vi "Process.vi"(8 "error in":errorcluster, 11 "Maui 2.0":refnum<class "Maui 2.0.lvclass">) -> (0 "error out":errorcluster, 3 "Maui 2.0 out":refnum<class "Maui 2.0.lvclass">)   [LabVIEW 2020, in "Maui 2.0.lvclass"]
doc: "---------------------------------------------------------------\nJKI State Machine Objects™\nhttp://jki.net/state-machine-objects/\nCopyright (C) 2005-2015, JKI <info@jki.net>\nALL RIGHTS RESERVED"
uses:
  Maui 2.0.lvclass
  C:/Program Files (x86)/National Instruments/LabVIEW 2020/vi.lib/JKI/JKI SMO/SMO/SMO.lvclass
  <vilib>/JKI/JKI SMO/SMO/Typedefs/Parent Call--Enum.ctl
  <vilib>/JKI/JKI SMO/SMO/SMO.lvclass
  Lifeguard/Lifeguard.lvclass
  Maui Manager/Maui Manager.lvclass
  Maui Manager/Maui Manager.lvclass/Maui Manager.ctl
  Maui Manager/Accessors/Write Processes.vi
  Maui Manager/Accessors/Write Panels.vi
panel:
  # "For instructions on how to use the JKI State Machine Objects, examples and video tutorials, visit:\nhttp://jki.net/state-machine-objects/\n\nJKI State Machine Objects™\nhttp://jki.net/state-machine-objects/\nCopyright (C) 2005-2015, JKI <info@jki.net>\nALL RIGHTS RESERVED"
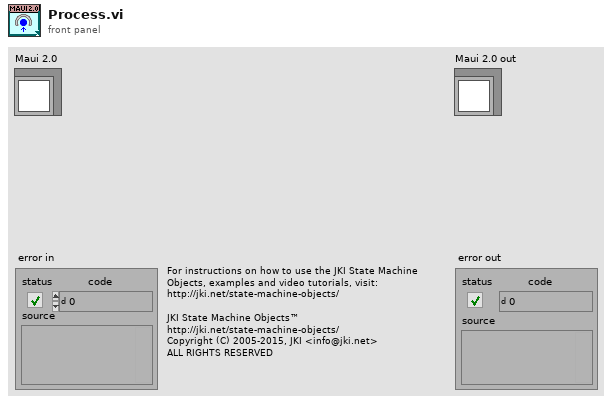
[diagram p1: front panel]
types:
  T1 = typedef "SMO.lvclass/Parent Call--Enum.ctl" = enum16{"Allows parent to run", "Does not request parent to run"}
  T2 = cluster{"Control":refnum<vi>, "Subpanel":refnum<vi>, "Active":i32, "Ctrl Class":string}
  T3 = enum32{"invalid app kind", "Development System", "Run Time System", "Student Edition", "Embedded LabVIEW", "Evaluation", "Custom"}
  T4 = enum32{"Invalid", "Standard", "Closed", "Hidden", "Minimized", "Maximized"}
  T5 = cluster{"Core":cluster{"Current VI Reference":refnum<vi>, "Close Panel on Exit?":bool, "error":errorcluster}, "Self Reference":refnum<class "Maui 2.0.lvclass">, "Subpanels":refnum<class "SMO.lvclass">[], "Panels":cluster{"Control":refnum<vi>, "Subpanel":refnum<vi>, "Active":i32, "Ctrl Class":string}[], "Lifeguard":refnum<class "Lifeguard.lvclass">, "Maui Manager":refnum<class "Maui Manager.lvclass">, "New Value":i32, "Panel":i32}
  T6 = typedef "Maui 2.0.lvclass/PrivateEvents--Maui 2.0.Set Panels.ctl" = cluster{"Control":refnum<vi>, "SubPnl":refnum<vi>}[]
  T7 = typedef "Maui 2.0.lvclass/PrivateEvents--Maui 2.0.Get Subpanels.ctl" = refnum<notifier>
  T8 = cluster{"Control":refnum<vi>, "Subpanel":refnum<vi>, "Active":i32, "Ctrl Class":string}[]
  T9 = cluster{"Current VI Reference":refnum<vi>, "Close Panel on Exit?":bool, "error":errorcluster}
  T10 = typedef "SMO.lvclass/Protected Events.ctl" = cluster{"StopProcesses":refnum<user-event>, "AbortProcesses":refnum<user-event>, "Config Changed":refnum<user-event>, "Dependency":refnum<user-event>}
  T11 = typedef "Maui 2.0.lvclass/PrivateEvents--Cluster.ctl" = cluster{"Set Subpanels":refnum<user-event>, "Get Subpanels":refnum<user-event>, "Set Panels":refnum<user-event>}
  T12 = typedef "Lifeguard.lvclass/PublicEvents--Cluster.ctl" = cluster{"New Panel Value":refnum<user-event>}
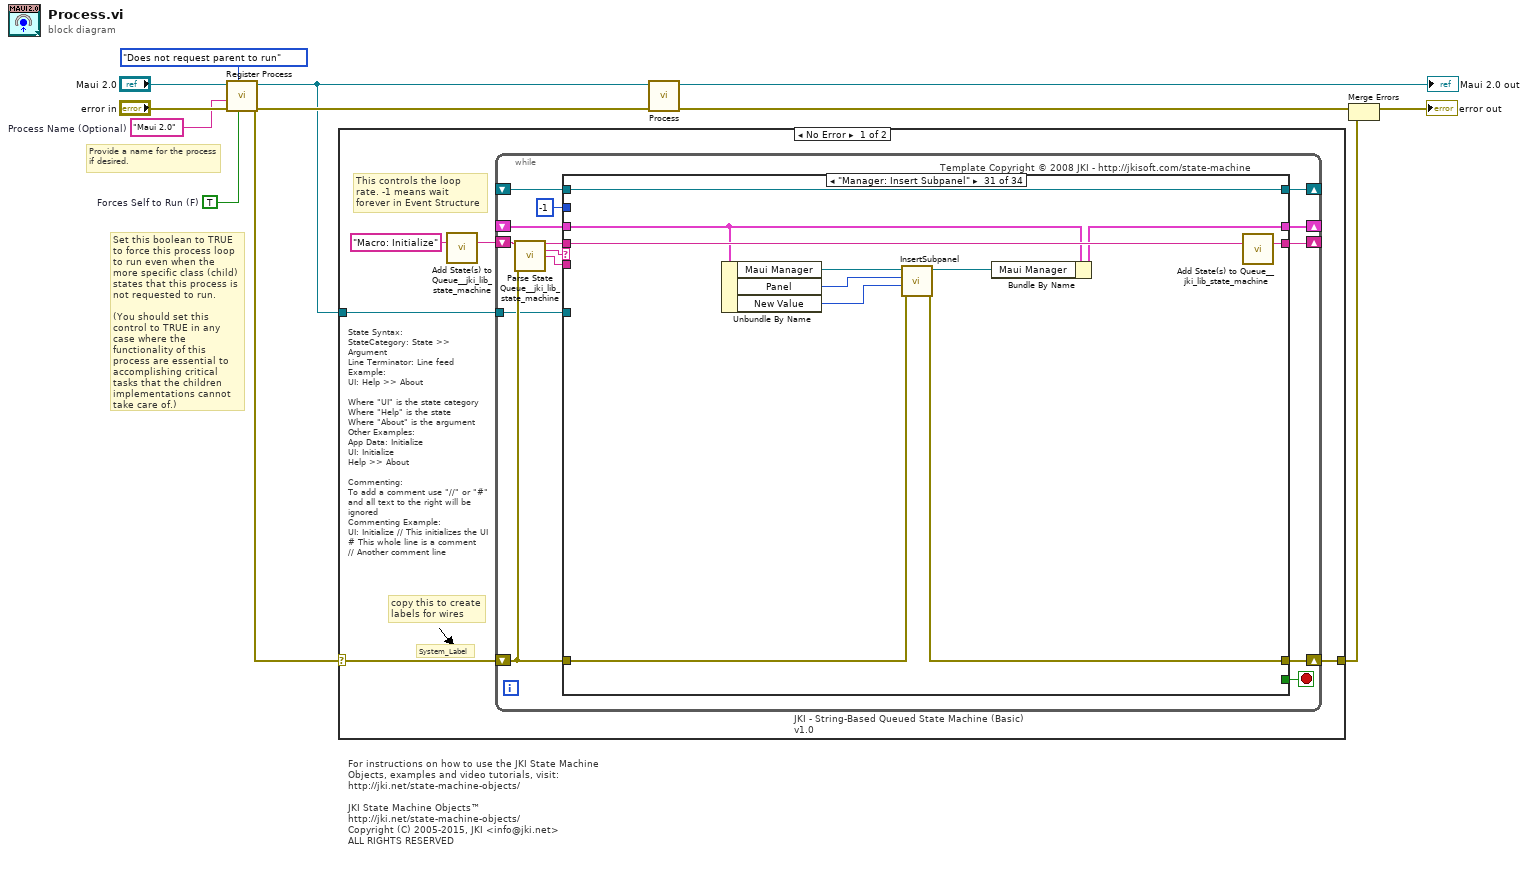
[diagram p0: block diagram]
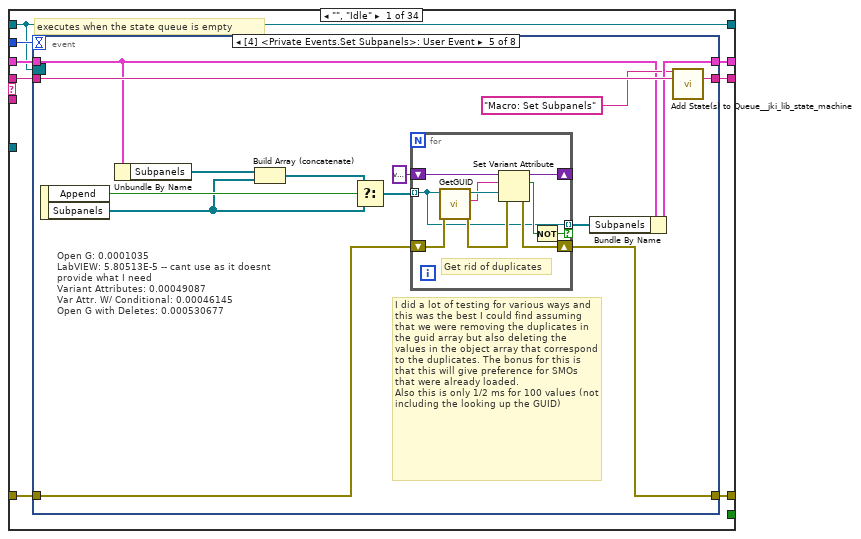
[diagram p2: hidden frame]
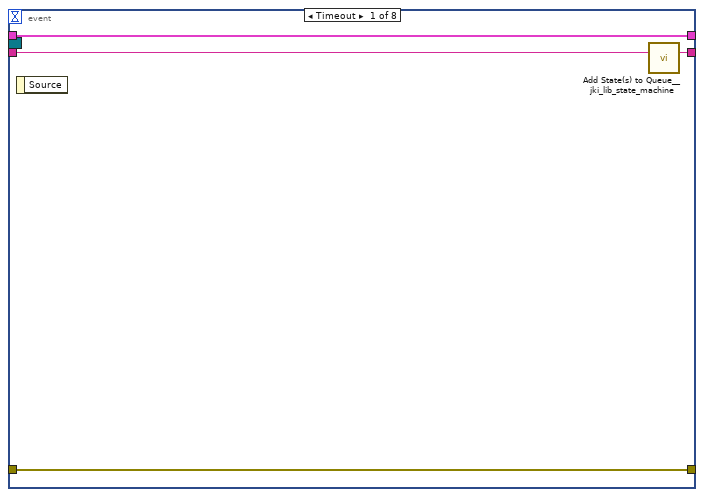
[diagram p3: hidden frame]
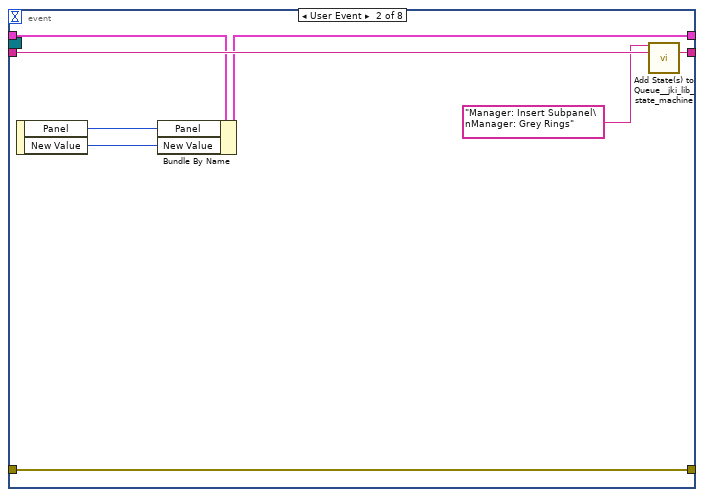
[diagram p4: hidden frame]
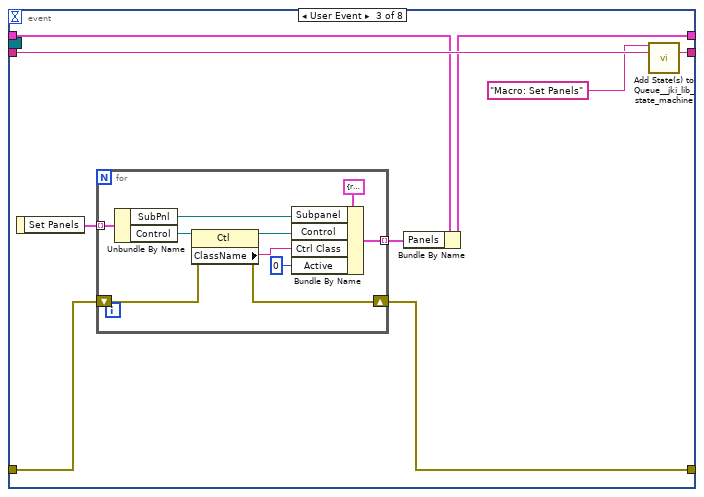
[diagram p5: hidden frame]
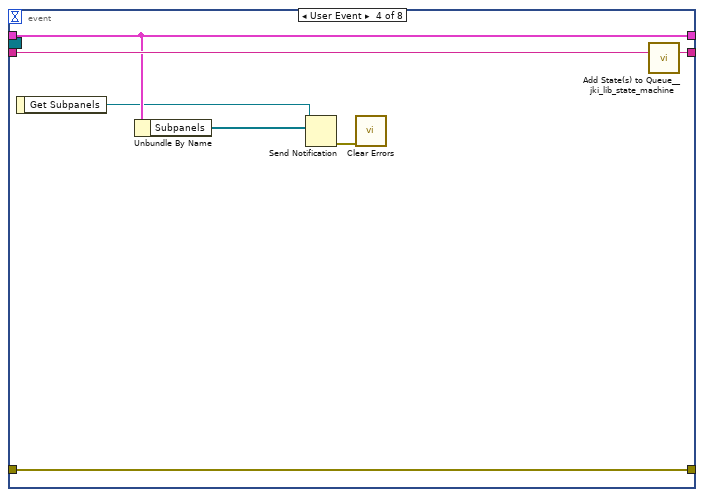
[diagram p6: hidden frame]
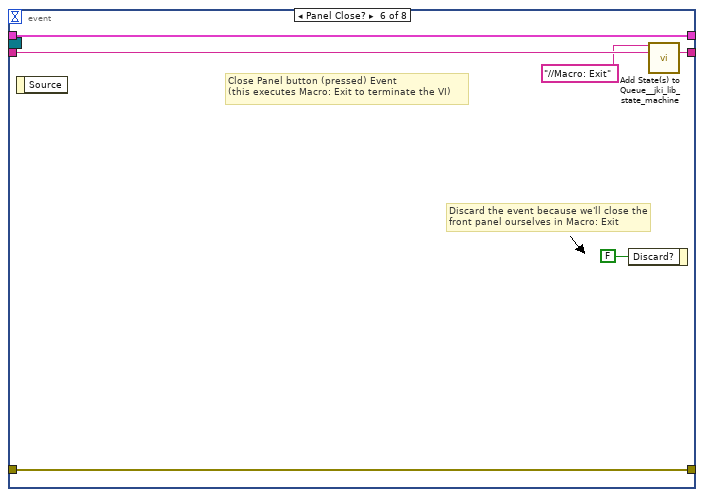
[diagram p7: hidden frame]
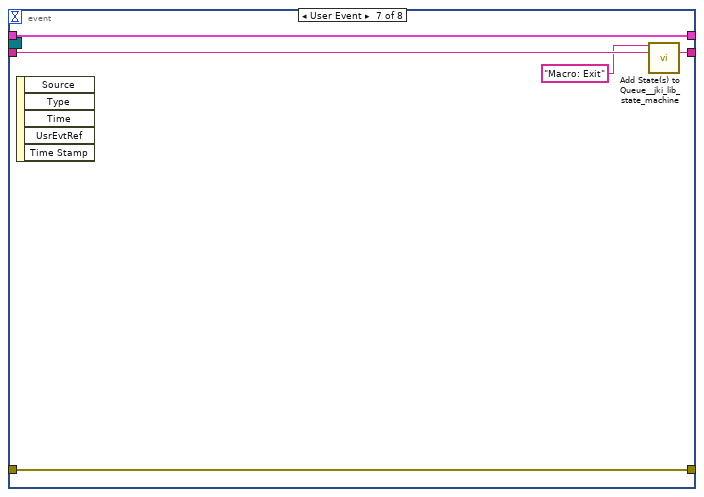
[diagram p8: hidden frame]
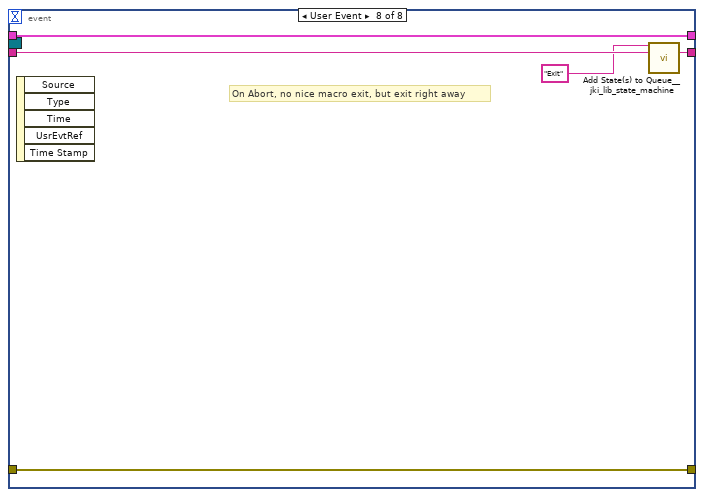
[diagram p9: hidden frame]
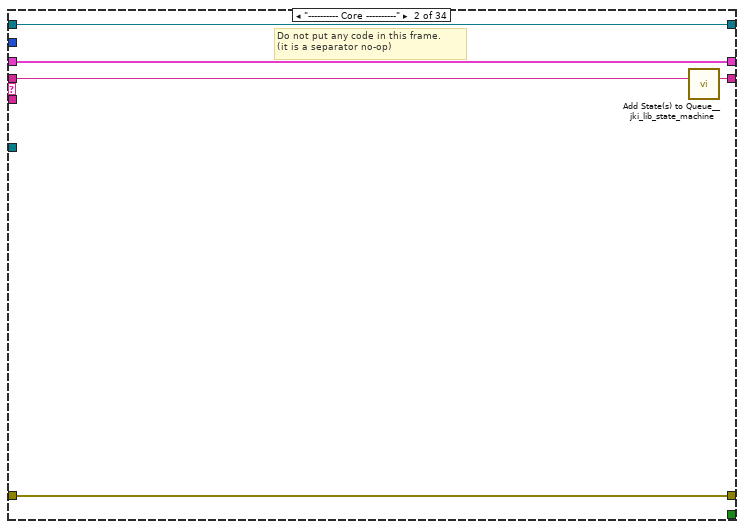
[diagram p10: hidden frame]
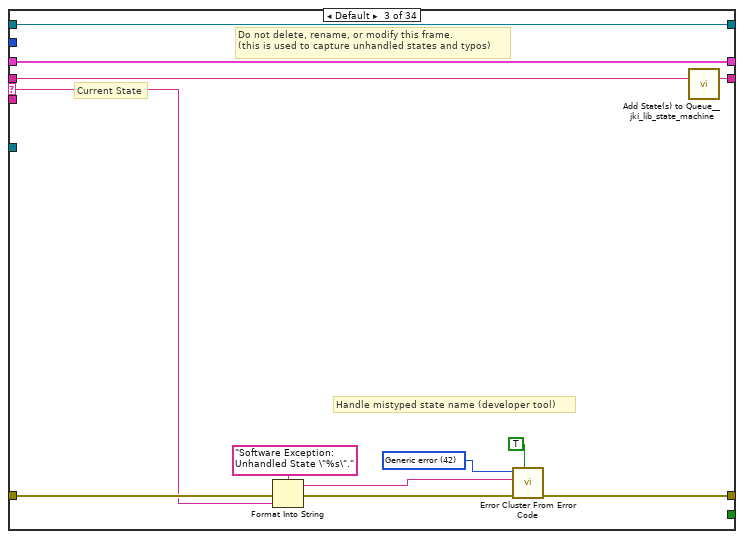
[diagram p11: hidden frame]
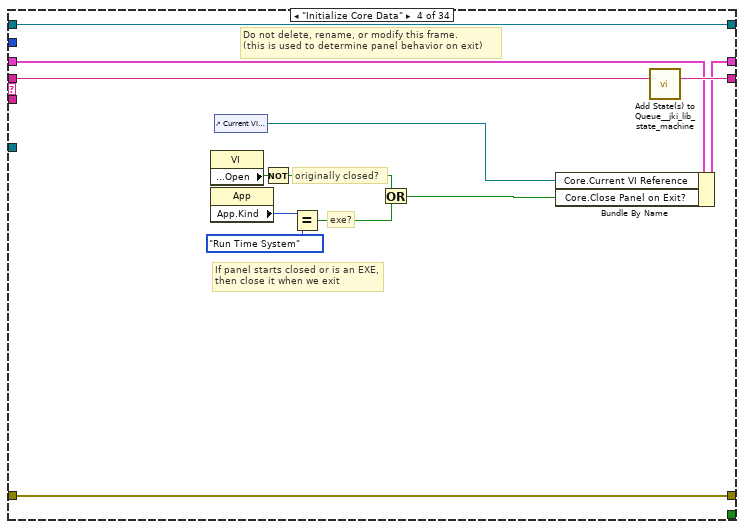
[diagram p12: hidden frame]
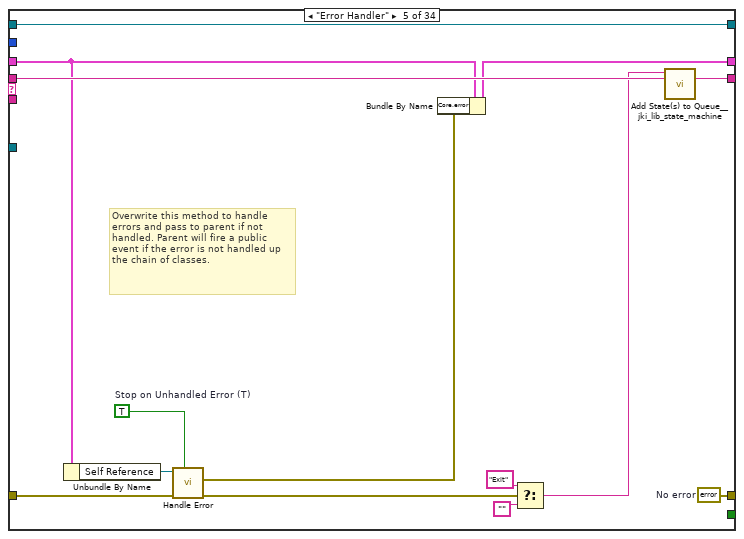
[diagram p13: hidden frame]
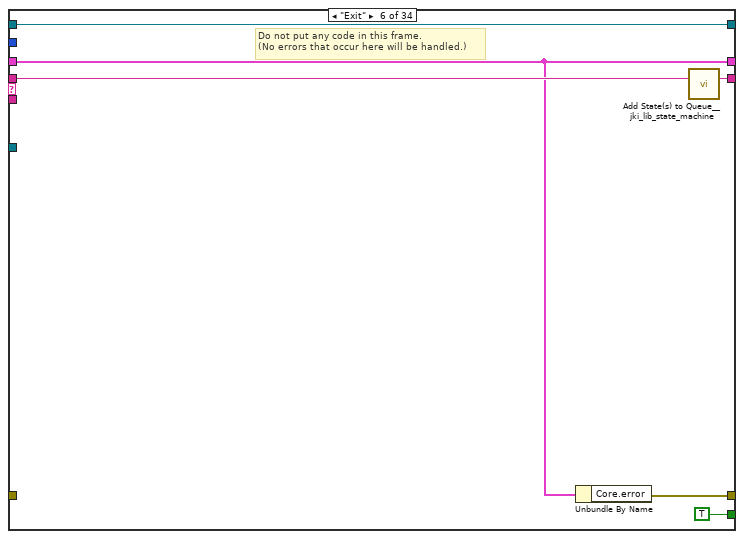
[diagram p14: hidden frame]
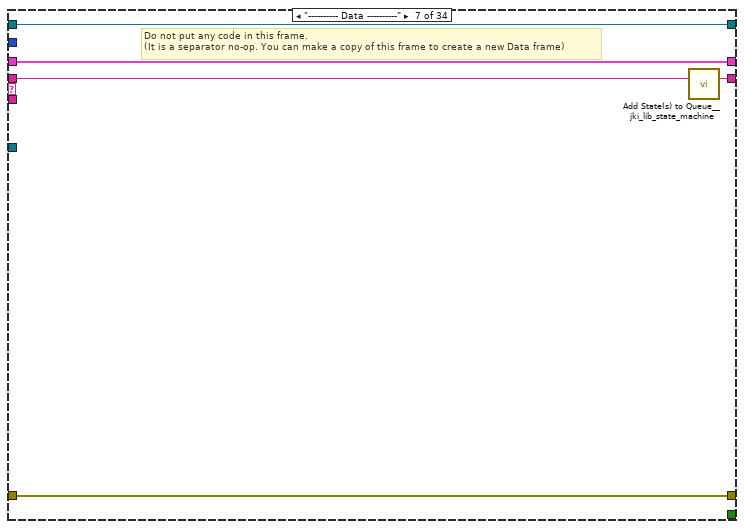
[diagram p15: hidden frame]
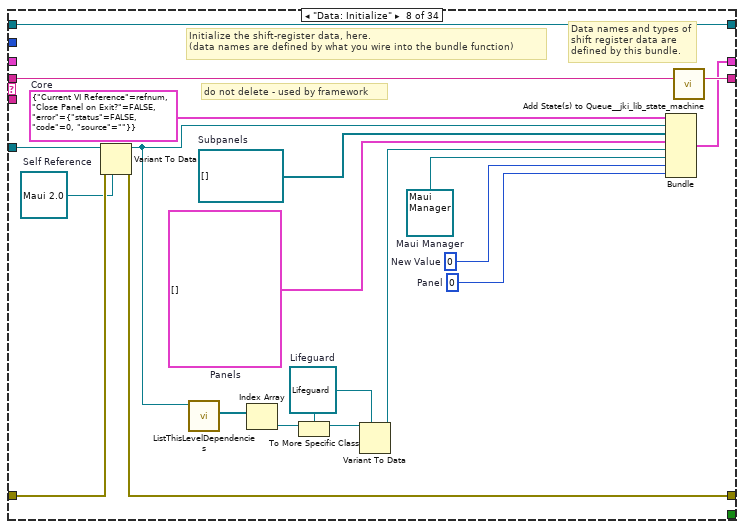
[diagram p16: hidden frame]
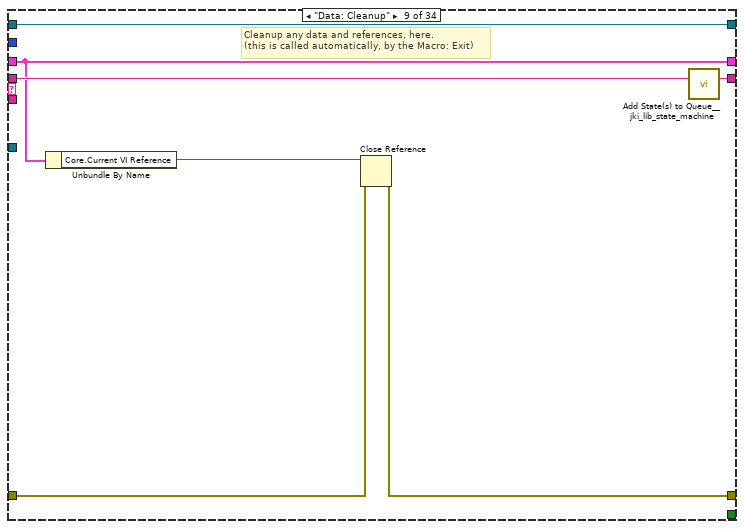
[diagram p17: hidden frame]
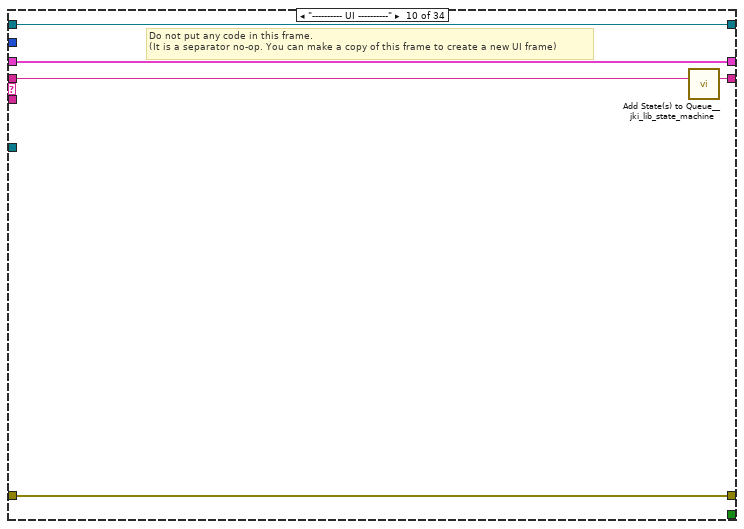
[diagram p18: hidden frame]
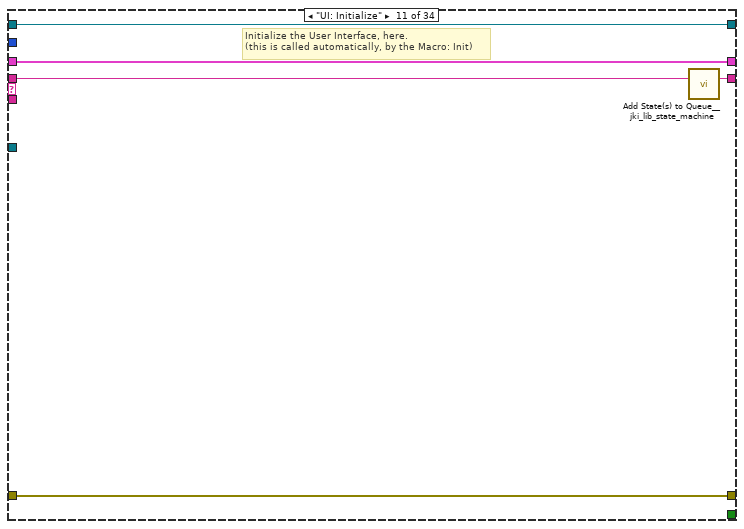
[diagram p19: hidden frame]
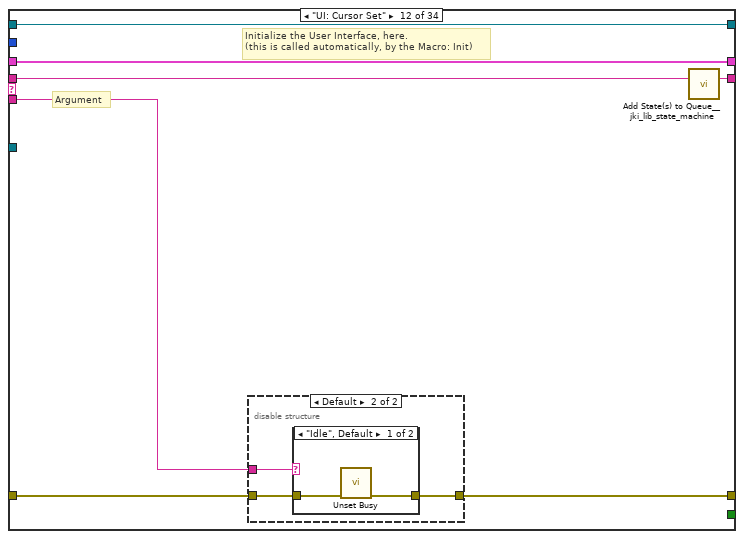
[diagram p20: hidden frame]
diagram:
  w2 = TRUE  # Forces Self to Run (F)
  w1 = "Maui 2.0"  # Process Name (Optional)
  # "Provide a name for the process\nif desired."
  # "Set this boolean to TRUE to force this process loop to run even when the more specific class (child) states that this process is not requested to run.\n\n(You should set this control to TRUE in any case where the functionality of this process are essential to accomplishing critical tasks that the children implementations cannot take care of.)"
  # "For instructions on how to use the JKI State Machine Objects, examples and video tutorials, visit:\nhttp://jki.net/state-machine-objects/\n\nJKI State Machine Objects™\nhttp://jki.net/state-machine-objects/\nCopyright (C) 2005-2015, JKI <info@jki.net>\nALL RIGHTS RESERVED"
  n1 = call <vilib>:"Register Process.vi"("Forces Self to Run (F)"=w2, "Parent Call"=Parent_Call--Enum."Does not request parent to run", "error in (no error)"="error in", "Process Name (optional)"=w1, "SMO"="Maui 2.0") -> ("error out"=w8:errorcluster, "SMO out"=w7:refnum<class "Maui 2.0.lvclass">)  [unwired: 5 in]
  n2 = case shown="No Error" w8 {
    selector: w8 -> [w13 w448]
    tunnel: w7 -> [w14 _]
    tunnel: [w12 w448] -> w4
    frame No Error {
      # "State Syntax:\nStateCategory: State >> Argument\nLine Terminator: Line feed\nExample:\nUI: Help >> About\n\nWhere \"UI\" is the state category\nWhere \"Help\" is the state\nWhere \"About\" is the argument\nOther Examples:\nApp Data: Initialize\nUI: Initialize\nHelp >> About\n\nCommenting:\nTo add a comment use \"//\" or \"#\" and all text to the right will be ignored\nCommenting Example:\nUI: Initialize // This initializes the UI\n# This whole line is a comment\n// Another comment line"
      # "copy this to create labels for wires"
      # "This controls the loop rate. -1 means wait forever in Event Structure"
      # "System_Label"
      n3 = call <vilib>:"Add State(s) to Queue__jki_lib_state_machine.vi"("State(s) in (\"\")"="Macro: Initialize") -> ("States Out"=w16:string)  [unwired: 14 in]
      n4 = while "JKI - String-Based Queued State Machine (Basic) v1.0" {
        shift-right: [w23] -> _
        shift-left: _ -> [w22]
        shift-right: [w26] -> w12
        shift-left: w13 -> [w20]
        shift-right: [w25] -> _
        shift-left: w16 -> [w27]
        tunnel: w14 -> [w19]
        shift-right: [w18] -> _
        shift-left: _ -> [w17]
        stop <- w24 stop-if-true
        # "Template Copyright © 2008 JKI - http://jkisoft.com/state-machine"
        n5 = call <vilib>:"Parse State Queue__jki_lib_state_machine.vi"("State Queue"=w27, "Error In (no error)"=w20) -> ("Remaining States"=w29:string, "Current State"=w30:string, "Arguments"=w28:string)  [unwired: 11 in]
        n6 = case shown="\"Manager: Insert Subpanel\"" w30 {
          selector: w30 -> [_ _ w123 _ _ _ _ _ _ _ _ _ _ _ _ _ _ _ _ _ _ _ _ _ _ _ _ _ _ _ _ _ _ _]
          tunnel: w29 -> [w38 w121 w127 w146 w160 w166 w171 w191 w198 w203 w208 w215 w231 w263 w268 w280 w292 w301 w315 w320 w331 w336 w351 w357 w364 w369 w376 w387 w396 w405 w416 w425 w437 w447]
          tunnel: w28 -> [_ _ _ _ _ _ _ _ _ _ _ w209 w225 _ _ _ _ _ _ _ _ _ _ _ _ _ _ _ _ _ _ _ _ _]
          tunnel: w22 -> [w36 w118 w125 w137 w154 w162 w168 _ w193 w200 w206 w213 w227 w260 w265 w272 w288 w297 w306 w317 w328 w333 w349 w355 w359 w365 w371 w383 w391 w401 w412 w421 w433 w443]
          tunnel: [w35 w119 w129 w143 w155 w161 w169 w187 w194 w201 w205 w210 w228 w261 w266 w278 w290 w299 w313 w318 w322 w334 w345 w353 w361 w366 w373 w378 w393 w398 w409 w418 w430 w438] -> w26
          tunnel: w20 -> [w34 w119 w128 w143 w156 _ w169 w188 w195 w201 w205 w211 w229 w261 w266 w278 w290 w299 w313 w318 w323 w334 w346 w353 w361 w366 w373 w377 w393 w397 w408 w417 w426 w439]
          tunnel: [w37 w120 w126 w145 w159 w165 w170 w190 w197 w202 w207 w214 w230 w262 w267 w279 w291 w300 w314 w319 w330 w335 w350 w356 w363 w368 w375 w386 w395 w404 w415 w424 w436 w446] -> w25
          tunnel: [_ _ _ _ _ TRUE _ _ _ _ _ _ _ _ _ _ _ _ _ _ _ _ _ _ _ _ _ _ _ _ _ _ _ _] -> w24
          tunnel: [w33 w118 w125 w144 w153 w162 w168 w189 w193 w200 w206 w213 w227 w260 w265 w272 w288 w297 w306 w317 w328 w333 w349 w355 w360 w365 w372 w384 w392 w402 w413 w422 w434 w444] -> w23
          tunnel: -1 ("Timeout") -> [w32 _ _ _ _ _ _ _ _ _ _ _ _ _ _ _ _ _ _ _ _ _ _ _ _ _ _ _ _ _ _ _ _ _]
          tunnel: w19 -> [_ _ _ _ _ _ _ w185 _ _ _ _ _ _ _ _ _ _ _ _ _ _ _ _ _ _ _ _ _ _ _ _ _ _]
          tunnel: [w31 w117 w122 w134 w158 w163 w167 w184 w192 w199 w204 w212 w224 w259 w264 w277 w289 w298 w307 w316 w329 w332 w348 w354 w362 w367 w374 w385 w394 w403 w414 w423 w435 w445] -> w18
          tunnel: w17 -> [w31 w117 w122 w134 w158 w163 w167 w184 w192 w199 w204 w212 w224 w259 w264 w277 w289 w298 w307 w316 w329 w332 _ w354 w362 w367 w374 w385 w394 w403 w414 w423 w435 w445]
          frame "", "Idle" {
            # "executes when the state queue is empty"
            n7 = event shown="[4] <Private Events.Set Subpanels>: User Event" {
              selector: w31 -> [_ _ _ _ _ _ _ _]
              dyn-events: _ -> [_ _ _ _ _ _ _ _]
              timeout: w32 -> [_ _ _ _ _ _ _ _]
              tunnel: w38 -> [w42 w50 w59 w76 w90 w106 w111 w116]
              tunnel: [w41 w49 w58 w75 w89 w105 w110 w115] -> w37
              tunnel: w36 -> [w40 w47 w53 w73 w77 w103 w108 w113]
              tunnel: [w39 w46 w52 w74 w81 w104 w109 w114] -> w35
              tunnel: w34 -> [w39 w46 w51 w74 w80 w104 w109 w114]
              tunnel: [w40 w48 w55 w73 w84 w103 w108 w113] -> w33
              event Timeout {
                n8 = event-data() -> ()  [unwired: 1 in, 1 out]
                n9 = call <vilib>:"Add State(s) to Queue__jki_lib_state_machine.vi"("State(s) in (\"\")"=w42) -> ("States Out"=w41:string)  [unwired: 14 in]
              }
              event User Event {
                n10 = event-data() -> ("Panel"=w45:i32, "New Value"=w44:i32)  [unwired: 1 in]
                n11 = Bundle By Name(cluster=w47, "Panel"=w45, "New Value"=w44) -> (w48:T5)
                n12 = call <vilib>:"Add State(s) to Queue__jki_lib_state_machine.vi"("State(s) in Front (\"\")"="Manager: Insert Subpanel\nManager: Grey Rings", "State(s) in (\"\")"=w50) -> ("States Out"=w49:string)  [unwired: 13 in]
              }
              event User Event {
                n13 = event-data() -> ("Set Panels"=w57:T6)  [unwired: 1 in]
                n14 = for {
                  tunnel: w57 -> [w69] mode=indexing
                  tunnel: [w63] -> w54 mode=indexing
                  shift-right: [w60] -> w52
                  shift-left: w51 -> [w61]
                  n15 = Unbundle By Name(w69) -> ("SubPnl"=w64:refnum<vi>, "Control"=w67:refnum<vi>)
                  n16 = property class="Ctl"(reference=w67, error in=w61) -> (reference out=w65:refnum<vi>, error out=w60:errorcluster, "ClassName"=w66:string)
                  n17 = Bundle By Name(cluster=T2 {"Control"=refnum, "Subpanel"=refnum, "Active"=0, "Ctrl Class"=""} ("Panel"), "Subpanel"=w64, "Control"=w65, "Ctrl Class"=w66, "Active"=0) -> (w63:T2)
                }
                n18 = Bundle By Name(cluster=w53, "Panels"=w54) -> (w55:T5)
                n19 = call <vilib>:"Add State(s) to Queue__jki_lib_state_machine.vi"("State(s) in Front (\"\")"="Macro: Set Panels", "State(s) in (\"\")"=w59) -> ("States Out"=w58:string)  [unwired: 13 in]
              }
              event User Event {
                n20 = event-data() -> ("Get Subpanels"=w71:T7)  [unwired: 1 in]
                n21 = Unbundle By Name(w73) -> ("Subpanels"=w72:refnum<class "SMO.lvclass">[])
                n22 = Send Notification(notification=w72, notifier=w71) -> (error out=w70:errorcluster)  [unwired: 1 in, 1 out]
                n23 = call <vilib>:"Clear Errors.vi"("error in (no error)"=w70) -> ()  [unwired: 5 in, 2 out]
                n24 = call <vilib>:"Add State(s) to Queue__jki_lib_state_machine.vi"("State(s) in (\"\")"=w76) -> ("States Out"=w75:string)  [unwired: 14 in]
              }
              event User Event {
                # "Open G: 0.0001035\nLabVIEW: 5.80513E-5 -- cant use as it doesnt provide what I need\nVariant Attributes: 0.00049087\nVar Attr. W/ Conditional: 0.00046145\nOpen G with Deletes: 0.000530677"
                # "I did a lot of testing for various ways and this was the best I could find assuming that we were removing the duplicates in the guid array but also deleting the values in the object array that correspond to the duplicates. The bonus for this is that this will give preference for SMOs that were already loaded.\nAlso this is only 1/2 ms for 100 values (not including the looking up the GUID)"
                n25 = event-data() -> ("Append"=w86:bool, "Subpanels"=w85:refnum<class "SMO.lvclass">[])  [unwired: 1 in]
                n26 = Unbundle By Name(w77) -> ("Subpanels"=w88:refnum<class "SMO.lvclass">[])
                n27 = Build Array (concatenate)(w88, w85) -> (w87:refnum<class "SMO.lvclass">[])
                n28 = Select(t=w87, s=w86, f=w85) -> (s? t:f=w83:refnum<class "SMO.lvclass">[])
                n29 = for {
                  tunnel: w83 -> [w92] mode=indexing
                  shift-right: [w99] -> _
                  shift-left: variant -> [w100]
                  tunnel: [w92] -> w82 mode=indexing if=w97
                  shift-right: [w93] -> w81
                  shift-left: w80 -> [w95]
                  # "Get rid of duplicates"
                  n30 = call <vilib>:"GetGUID.vi"("error in (no error)"=w95, "SMO"=w92) -> ("error out"=w94:errorcluster, "GUID"=w91:string, "SMO out"=w98:refnum<class "SMO.lvclass">)  [unwired: 7 in]
                  n31 = Set Variant Attribute(Variant=w100, name=w91, value=w98, error in=w94) -> (Variant out=w99:variant, replaced=w96:bool, error out=w93:errorcluster)
                  n32 = Not(x=w96) -> (.not. x?=w97:bool)
                }
                n33 = Bundle By Name(cluster=w77, "Subpanels"=w82) -> (w84:T5)
                n34 = call <vilib>:"Add State(s) to Queue__jki_lib_state_machine.vi"("State(s) in Front (\"\")"="Macro: Set Subpanels", "State(s) in (\"\")"=w90) -> ("States Out"=w89:string)  [unwired: 13 in]
              }
              event Panel Close? {
                # "Discard the event because we'll close the front panel ourselves in Macro: Exit"
                # "Close Panel button (pressed) Event\n(this executes Macro: Exit to terminate the VI)"
                n35 = event-data() -> ()  [unwired: 1 in, 1 out]
                n36 = event-data ("Event Filter Node")("Discard?"=FALSE) -> ()  [unwired: 1 in, 1 out]
                n37 = call <vilib>:"Add State(s) to Queue__jki_lib_state_machine.vi"("State(s) in Front (\"\")"="//Macro: Exit", "State(s) in (\"\")"=w106) -> ("States Out"=w105:string)  [unwired: 13 in]
              }
              event User Event {
                n38 = event-data() -> ()  [unwired: 1 in, 5 out]
                n39 = call <vilib>:"Add State(s) to Queue__jki_lib_state_machine.vi"("State(s) in Front (\"\")"="Macro: Exit", "State(s) in (\"\")"=w111) -> ("States Out"=w110:string)  [unwired: 13 in]
              }
              event User Event {
                # "On Abort, no nice macro exit, but exit right away"
                n40 = event-data() -> ()  [unwired: 1 in, 5 out]
                n41 = call <vilib>:"Add State(s) to Queue__jki_lib_state_machine.vi"("State(s) in Front (\"\")"="Exit", "State(s) in (\"\")"=w116) -> ("States Out"=w115:string)  [unwired: 13 in]
              }
            }
          }
          frame "---------- Core ----------" {
            # "Do not put any code in this frame.\n(it is a separator no-op)"
            n42 = call <vilib>:"Add State(s) to Queue__jki_lib_state_machine.vi"("State(s) in (\"\")"=w121) -> ("States Out"=w120:string)  [unwired: 14 in]
          }
          frame Default {
            w132 = 42 items=["No error", "Argument error", "Memory is full", "Out of zone", "End of file", "File already open", "Generic file I/O error", "File not found", "File permission error", "Disk is full", "Duplicate path", "Too many files open", "System feature not enabled", "Resource file not found", "Cannot add resource", "Resource not found", "Image not found", "Image memory error", "Pen does not exist", "Config type invalid", "Config token not found", "Config parse error", "Config memory error", "Bad external code format", "Bad external code offset", "External code not present", "Null window", "Destroy window error", "Null menu", "Print aborted", "Bad print record", "Print driver error", "Windows error during printing", "Memory error during printing", "Print dialog error", "Generic print error", "Invalid device refnum", "Device not found", "Device parameter error", "Device unit error", "Cannot open device", "Device call aborted", "Generic error", "Cancelled by user", "Object ID too low", "Object ID too high", "Object not in heap", "Unknown heap", "Unknown object (invalid DefProc)", "Unknown object (DefProc not in table)", "Message out of range", "Invalid (null) method", "Unknown message", "Manager call not supported", "Bad address", "Network operation in progress", "Network operation timed out", "Connection is busy", "Network attribute not supported", "Network error", "Address in use", "System out of memory", "Connection aborted", "Connection refused", "Not connected", "Already connected", "Connection closed", "Initialization error (interapplication manager)", "Bad occurrence", "Wait on unbound occurrence handler", "Occurrence queue overflow", "Datalog type conflict", "Unused", "Unrecognized type (interapplication manager)", "Memory corrupt", "Failed to make temporary DLL", "Old CIN version", "Drag socket not found", "Failed to load drop-object", "Failed to register OLE object", "Failed to release OLE object", "Format specifier type mismatch", "Unknown format specifier", "Too few format specifiers", "Too many format specifiers", "Scan failed", "Newer CIN version", "Error converting to variant", "Runtime menu error", "Password tampered", "Variant attribute not found", "Incompatible variant data type", "Event data is not available", "Event Store is not present", "Occurrence is not found", "Event Queue is not created", "Event info is not available", "Refnum passed is NULL", "Error retrieving Class GUID", "Error retrieving CoClass GUID", "Error retrieving TypeLib GUID.", "Bad built application magic bytes.", "Specific driver is different from the specific driver associated with the Logical Name.", "There is no session opened to the class driver.", "Max Error", "MAX - Error with config objects", "MAX - Error loading configuration", "MAX - Group not supported"]
            # "Current State"
            # "Do not delete, rename, or modify this frame.\n(this is used to capture unhandled states and typos)"
            # "Handle mistyped state name (developer tool)"
            n43 = Format Into String(format string="Software Exception: Unhandled State \"%s\"." ("message"), error in=w128, w123) -> (resulting string=w131:string, error out=w130:errorcluster)  [unwired: 1 in]
            n44 = call <vilib>:"Error Cluster From Error Code.vi"("show call chain? (False)"=TRUE, "error in (no error)"=w130, "error message (\"\")"=w131, "error code (0)"=w132) -> ("error out"=w129:errorcluster)  [unwired: 5 in]
            n45 = call <vilib>:"Add State(s) to Queue__jki_lib_state_machine.vi"("State(s) in (\"\")"=w127) -> ("States Out"=w126:string)  [unwired: 14 in]
          }
          frame "Initialize Core Data" {
            # "Do not delete, rename, or modify this frame.\n(this is used to determine panel behavior on exit)"
            # "originally closed?"
            # "exe?"
            # "If panel starts closed or is an EXE, then close it when we exit"
            n46 = property on="Property Node" class="VI"() -> ("Front Panel.Open"=w142:bool)  [unwired: 2 in, 2 out]
            n47 = property on="Property Node" class="App"() -> ("App.Kind"=w141:T3)  [unwired: 2 in, 2 out]
            n48 = control-ref of="Current VI Reference"() -> (w135:refnum<vi>)
            n49 = Not(x=w142) -> (.not. x?=w139:bool)
            n50 = Equal?(x=w141, y=T3."Run Time System" ("Application:Kind")) -> (x = y?=w138:bool)
            n51 = Or(x=w139, y=w138) -> (x .or. y?=w136:bool)
            n52 = Bundle By Name(cluster=w137, "Core.Current VI Reference"=w135, "Core.Close Panel on Exit?"=w136) -> (w144:T5)
            n53 = call <vilib>:"Add State(s) to Queue__jki_lib_state_machine.vi"("State(s) in (\"\")"=w146) -> ("States Out"=w145:string)  [unwired: 14 in]
          }
          frame "Error Handler" {
            w147 = TRUE  # Stop on Unhandled Error (T)
            w155 = errorcluster {"status"=FALSE, "code"=0, "source"=""}  # No error
            # "Overwrite this method to handle errors and pass to parent if not handled. Parent will fire a public event if the error is not handled up the chain of classes."
            n54 = Unbundle By Name(w154) -> ("Self Reference"=w157:refnum<class "Maui 2.0.lvclass">)
            n55 = call-dynamic "Handle Error.vi"("Stop on Unhandled Error (T)"=w147, "error in"=w156, "SMO"=w157) -> ("handling error"=w148:errorcluster, "Unhandled error"=w151:errorcluster)  [unwired: 6 in, 1 out]
            n56 = Bundle By Name(cluster=w154, "Core.error"=w151) -> (w153:T5)
            n57 = Select(t="Exit", s=w148, f="" ("Empty String Constant")) -> (s? t:f=w152:string)
            n58 = call <vilib>:"Add State(s) to Queue__jki_lib_state_machine.vi"("State(s) in Front (\"\")"=w152, "State(s) in (\"\")"=w160) -> ("States Out"=w159:string)  [unwired: 13 in]
          }
          frame "Exit" {
            # "Do not put any code in this frame.\n(No errors that occur here will be handled.)"
            n59 = Unbundle By Name(w162) -> ("Core.error"=w161:errorcluster)
            n60 = call <vilib>:"Add State(s) to Queue__jki_lib_state_machine.vi"("State(s) in (\"\")"=w166) -> ("States Out"=w165:string)  [unwired: 14 in]
          }
          frame "---------- Data ----------" {
            # "Do not put any code in this frame.\n(It is a separator no-op. You can make a copy of this frame to create a new Data frame)"
            n61 = call <vilib>:"Add State(s) to Queue__jki_lib_state_machine.vi"("State(s) in (\"\")"=w171) -> ("States Out"=w170:string)  [unwired: 14 in]
          }
          frame "Data: Initialize" {
            w173 = 0  # New Value
            w172 = 0  # Panel
            w174 = refnum<class "Maui Manager.lvclass"> refnum  # Maui Manager
            w176 = refnum<class "Lifeguard.lvclass"> refnum  # Lifeguard
            w181 = T8 []  # Panels
            w182 = refnum<class "SMO.lvclass">[] []  # Subpanels
            w183 = T9 {"Current VI Reference"=refnum, "Close Panel on Exit?"=FALSE, "error"={"status"=FALSE, "code"=0, "source"=""}}  # Core
            w186 = refnum<class "Maui 2.0.lvclass"> refnum  # Self Reference
            # "do not delete - used by framework"
            # "Data names and types of shift register data are defined by this bundle."
            # "Initialize the shift-register data, here.\n(data names are defined by what you wire into the bundle function)"
            n62 = Variant To Data(error in=w188, type=w186, Variant=w185) -> (data=w178:refnum<class "Maui 2.0.lvclass">, error out=w187:errorcluster)
            n63 = call <vilib>:"ListThisLevelDependencies.vi"("SMO in"=w178) -> ("[My Dependencies]"=w180:refnum<class "SMO.lvclass">[])  [unwired: 8 in, 2 out]
            n64 = Index Array(array=w180) -> (element=w179:refnum<class "SMO.lvclass">)  [unwired: 1 in]
            n65 = To More Specific Class(target class=w176, reference=w179) -> (specific class reference=w177:refnum<class "Lifeguard.lvclass">)  [unwired: 1 in, 1 out]
            n66 = Variant To Data(type=w176, Variant=w177) -> (data=w175:refnum<class "Lifeguard.lvclass">)  [unwired: 1 in, 1 out]
            n67 = Bundle("Core"=w183, "Self Reference"=w178, "Subpanels"=w182, "Panels"=w181, "Lifeguard"=w175, "Maui Manager"=w174, "New Value"=w173, "Panel"=w172) -> (w189:T5)  [unwired: 1 in]
            n68 = call <vilib>:"Add State(s) to Queue__jki_lib_state_machine.vi"("State(s) in (\"\")"=w191) -> ("States Out"=w190:string)  [unwired: 14 in]
          }
          frame "Data: Cleanup" {
            # "Cleanup any data and references, here.\n(this is called automatically, by the Macro: Exit)"
            n69 = Unbundle By Name(w193) -> ("Core.Current VI Reference"=w196:refnum<vi>)
            n70 = Close Reference(reference=w196, error in (no error)=w195) -> (error out=w194:errorcluster)
            n71 = call <vilib>:"Add State(s) to Queue__jki_lib_state_machine.vi"("State(s) in (\"\")"=w198) -> ("States Out"=w197:string)  [unwired: 14 in]
          }
          frame "---------- UI ----------" {
            # "Do not put any code in this frame.\n(It is a separator no-op. You can make a copy of this frame to create a new UI frame)"
            n72 = call <vilib>:"Add State(s) to Queue__jki_lib_state_machine.vi"("State(s) in (\"\")"=w203) -> ("States Out"=w202:string)  [unwired: 14 in]
          }
          frame "UI: Initialize" {
            # "Initialize the User Interface, here.\n(this is called automatically, by the Macro: Init)"
            n73 = call <vilib>:"Add State(s) to Queue__jki_lib_state_machine.vi"("State(s) in (\"\")"=w208) -> ("States Out"=w207:string)  [unwired: 14 in]
          }
          frame "UI: Cursor Set" {
            # "Argument"
            # "Initialize the User Interface, here.\n(this is called automatically, by the Macro: Init)"
            n74 = disable-structure "Conditional Disable Structure" shown="Default" {
              disable-tunnel: w211 -> [w216 w219]
              disable-tunnel: [w216 w218] -> w210
              disable-tunnel: w209 -> [_ w217]
              frame condition #0 {
              }
              frame condition #1 (active) {
                n75 = case shown="\"Idle\", Default" w217 {
                  tunnel: w219 -> [w221 w223]
                  tunnel: [w220 w222] -> w218
                  frame "Idle", Default {
                    n76 = call <vilib>:"Unset Busy.vi"("error in (no error)"=w221) -> ("error out"=w220:errorcluster)  [unwired: 10 in]
                  }
                  frame "Busy" {
                    n77 = call <vilib>:"Set Busy.vi"("error in (no error)"=w223) -> ("error out"=w222:errorcluster)  [unwired: 9 in, 1 out]
                  }
                }
              }
            }
            n78 = call <vilib>:"Add State(s) to Queue__jki_lib_state_machine.vi"("State(s) in (\"\")"=w215) -> ("States Out"=w214:string)  [unwired: 14 in]
          }
          frame "UI: Front Panel State" {
            # "Argument"
            # "Set Front Panel Open or Closed\n(Usage: \"UI: Front Panel State >> Open|Close\")"
            n79 = Unbundle By Name(w227) -> ("Core.Current VI Reference"=w226:refnum<vi>)
            n80 = disable-structure "Conditional Disable Structure" shown="Default" {
              disable-tunnel: w229 -> [w235 w258]
              disable-tunnel: [w234 w258] -> w228
              disable-tunnel: w226 -> [w233 _]
              disable-tunnel: w225 -> [w232 _]
              frame condition #0 (active) {
                n81 = case shown="\"Close\"" w232 {
                  tunnel: w235 -> [w239 w252]
                  tunnel: [w241 w253] -> w234
                  tunnel: w233 -> [w240 w250]
                  frame "Open", Default {
                    n82 = property on="Property Node" class="VI"(reference=w240, error in=w239) -> (reference out=w237:refnum<vi>, error out=w238:errorcluster, "FP.State"=w236:T4)
                    n83 = case shown="\"Closed\"" w236 {
                      tunnel: [w244 w247] -> w241
                      tunnel: w238 -> [w243 w247]
                      tunnel: w237 -> [w242 _]
                      frame "Closed" {
                        n84 = invoke on="Invoke Node" class="VI" method="FP.Open"(reference=w242, error in=w243, "Activate"=TRUE, "State"=T4."Standard") -> (error out=w244:errorcluster)  [unwired: 1 in, 4 out]
                      }
                      frame Default {
                      }
                    }
                  }
                  frame "Close" {
                    n85 = property on="Property Node" class="VI"(reference=w250, error in=w252) -> (reference out=w249:refnum<vi>, error out=w251:errorcluster, "FP.State"=w248:T4)
                    n86 = case shown="Default" w248 {
                      tunnel: [w254 w257] -> w253
                      tunnel: w251 -> [w254 w256]
                      tunnel: w249 -> [_ w255]
                      frame "Invalid", "Closed" {
                      }
                      frame Default {
                        n87 = invoke on="Invoke Node" class="VI" method="FP.Close"(reference=w255, error in=w256) -> (error out=w257:errorcluster)  [unwired: 1 in, 2 out]
                      }
                    }
                  }
                }
              }
              frame condition #1 {
              }
            }
            n88 = call <vilib>:"Add State(s) to Queue__jki_lib_state_machine.vi"("State(s) in (\"\")"=w231) -> ("States Out"=w230:string)  [unwired: 14 in]
          }
          frame "---------- Macro ----------" {
            # "Do not put any code in this frame.\n(It is a separator no-op. You can make a copy of this frame to create a new Macro frame)"
            n89 = call <vilib>:"Add State(s) to Queue__jki_lib_state_machine.vi"("State(s) in (\"\")"=w263) -> ("States Out"=w262:string)  [unwired: 14 in]
          }
          frame "Macro: New Panel Value" {
            # "Do not put any code in this frame.\n(It is a separator no-op. You can make a copy of this frame to create a new Macro frame)"
            n90 = call <vilib>:"Add State(s) to Queue__jki_lib_state_machine.vi"("State(s) in (\"\")"=w268) -> ("States Out"=w267:string)  [unwired: 14 in]
          }
          frame "Macro: Set Panels" {
            # "Still notify lifeguard of the change"
            # "Do nothing if there isnt any subpanels yet."
            # "Do not put any code in this frame.\n(It is a separator no-op. You can make a copy of this frame to create a new Macro frame)"
            n91 = Unbundle By Name(w272) -> ("Subpanels"=w271:refnum<class "SMO.lvclass">[])
            n92 = Empty Array?(array=w271) -> (empty?=w276:bool)
            n93 = Select(t="", s=w276, f="Action: Populate Panels\nManager: Initialize Panels") -> (s? t:f=w273:string)
            n94 = call <vilib>:"Add State(s) to Queue__jki_lib_state_machine.vi"("State(s) in Front (\"\")"="Lifeguard: New Panels\nManager: Set Panels", "State(s) in (\"\")"=w273) -> ("States Out"=w269:string)  [unwired: 13 in]
            n95 = call <vilib>:"Add State(s) to Queue__jki_lib_state_machine.vi"("State(s) in Front (\"\")"=w269, "State(s) in (\"\")"=w280) -> ("States Out"=w279:string)  [unwired: 13 in]
          }
          frame "Macro: Set Subpanels" {
            # "If there is no panels, we dont want to try and do anything yet."
            # "Called on Set Subpanels Event. \n(Checks the state of the subpanels, and the controls and decides what to do)"
            n96 = Unbundle By Name(w288) -> ("Panels"=w287:T8)
            n97 = Empty Array?(array=w287) -> (empty?=w286:bool)
            n98 = Select(t="", s=w286, f="Action: Populate Panels\nManager: Initialize Panels") -> (s? t:f=w283:string)
            n99 = call <vilib>:"Add State(s) to Queue__jki_lib_state_machine.vi"("State(s) in Front (\"\")"="Manager: Set Subpanels" ("State(s) in Front (\"\")"), "State(s) in (\"\")"=w283) -> ("States Out"=w281:string)  [unwired: 13 in]
            n100 = call <vilib>:"Add State(s) to Queue__jki_lib_state_machine.vi"("State(s) in Front (\"\")"=w281, "State(s) in (\"\")"=w292) -> ("States Out"=w291:string)  [unwired: 13 in]
          }
          frame "Macro: Initialize" {
            w295 = "//UI: Initialize\n//UI: Front Panel State >> Open"  # //UI: Initialize //UI: Front Panel State >> Open
            # "Initialization Macro\n(This is called once, when the VI starts)"
            n101 = call <vilib>:"Add State(s) to Queue__jki_lib_state_machine.vi"("State(s) in Front (\"\")"="Data: Initialize\nInitialize Core Data\nEvents: Register", "State(s) in (\"\")"="Process: Sync", "State(s) at Back (\"\")"=w295) -> ("States Out"=w294:string)  [unwired: 12 in]
            n102 = call <vilib>:"Add State(s) to Queue__jki_lib_state_machine.vi"("State(s) in Front (\"\")"=w294, "State(s) in (\"\")"=w301) -> ("States Out"=w300:string)  [unwired: 13 in]
          }
          frame "Macro: Exit" {
            # "Exit Macro\n(This is called once, when the VI exits)"
            n103 = Unbundle By Name(w306) -> ("Core.Close Panel on Exit?"=w312:bool)
            n104 = Select(t="UI: Front Panel State >> Close", s=w312, f="" ("Empty String Constant")) -> (s? t:f=w309:string)
            n105 = call <vilib>:"Add State(s) to Queue__jki_lib_state_machine.vi"("State(s) in Front (\"\")"="Data: Cleanup\nEvents: Unregister", "State(s) in (\"\")"="Process: Sync", "State(s) at Back (\"\")"="Exit") -> ("States Out"=w303:string)  [unwired: 12 in]
            n106 = call <vilib>:"Add State(s) to Queue__jki_lib_state_machine.vi"("State(s) in (\"\")"=w309, "State(s) at Back (\"\")"=w303) -> ("States Out"=w308:string)  [unwired: 13 in]
            n107 = call <vilib>:"Add State(s) to Queue__jki_lib_state_machine.vi"("State(s) in Front (\"\")"=w308, "State(s) in (\"\")"=w315) -> ("States Out"=w314:string)  [unwired: 13 in]
          }
          frame "---------- Process ----------" {
            # "Template Separator\n(You can make a copy of, or modify, this frame)"
            n108 = call <vilib>:"Add State(s) to Queue__jki_lib_state_machine.vi"("State(s) in (\"\")"=w320) -> ("States Out"=w319:string)  [unwired: 14 in]
          }
          frame "Process: Sync" {
            n109 = Unbundle By Name(w328) -> ("Self Reference"=w324:refnum<class "Maui 2.0.lvclass">)
            n110 = call <vilib>:"WaitOnProcessSync.vi"("error in (no error)"=w323, "SMO"=w324) -> ("error out"=w322:errorcluster, "Don't run?"=w327:bool)  [unwired: 7 in, 1 out]
            n111 = Select(t="Data: Cleanup\nEvents: Unregister\nExit", s=w327, f="" ("Empty String Constant")) -> (s? t:f=w321:string)
            n112 = call <vilib>:"Add State(s) to Queue__jki_lib_state_machine.vi"("State(s) in Front (\"\")"=w321, "State(s) in (\"\")"=w331) -> ("States Out"=w330:string)  [unwired: 13 in]
          }
          frame "---------- Events ----------" {
            # "Template Separator\n(You can make a copy of, or modify, this frame)"
            n113 = call <vilib>:"Add State(s) to Queue__jki_lib_state_machine.vi"("State(s) in (\"\")"=w336) -> ("States Out"=w335:string)  [unwired: 14 in]
          }
          frame "Events: Register" {
            # "Expand to add\nmore events"
            n114 = Unbundle By Name(w349) -> ("Self Reference"=w343:refnum<class "Maui 2.0.lvclass">, "Lifeguard"=w342:refnum<class "Lifeguard.lvclass">)
            n115 = call <vilib>:"GetProtectedEvents.vi"("SMO"=w343) -> ("error out"=w341:errorcluster, "SMO Protected Events"=w347:T10)  [unwired: 8 in, 1 out]
            n116 = call "Maui 2.0.GetPrivateEvents.vi"("Maui 2.0"=w343) -> ("error out"=w340:errorcluster, "Private Events"=w338:T11)  [unwired: 8 in, 1 out]
            n117 = call "Lifeguard.GetPublicEvents.vi"("Lifeguard"=w342) -> ("error out"=w339:errorcluster, "Public Events"=w337:T12)  [unwired: 8 in, 1 out]
            n118 = register-events(w347, w338, w337) -> (reference out=w348:refnum<event-registration>, error out=w344:errorcluster)  [unwired: 2 in]
            n119 = Merge Errors(w346, w344, w341, w340, w339) -> (w345:errorcluster)
            n120 = call <vilib>:"Add State(s) to Queue__jki_lib_state_machine.vi"("State(s) in (\"\")"=w351) -> ("States Out"=w350:string)  [unwired: 14 in]
          }
          frame "Events: Unregister" {
            n121 = Unregister For Events(event registration refnum=w354, error in=w353) -> (error out=w352:errorcluster)
            n122 = call <vilib>:"Clear Errors.vi"("error in (no error)"=w352) -> ()  [unwired: 5 in, 2 out]
            n123 = call <vilib>:"Add State(s) to Queue__jki_lib_state_machine.vi"("State(s) in (\"\")"=w357) -> ("States Out"=w356:string)  [unwired: 14 in]
          }
          frame "---------- Action ----------" {
            n124 = Unbundle By Name(w359) -> ("Self Reference"=w358:refnum<class "Maui 2.0.lvclass">)
            n125 = Bundle By Name(cluster=w359, "Self Reference"=w358) -> (w360:T5)
            n126 = call <vilib>:"Add State(s) to Queue__jki_lib_state_machine.vi"("State(s) in (\"\")"=w364) -> ("States Out"=w363:string)  [unwired: 14 in]
          }
          frame "Action: Populate Panels" {
            n127 = call <vilib>:"Add State(s) to Queue__jki_lib_state_machine.vi"("State(s) in (\"\")"=w369) -> ("States Out"=w368:string)  [unwired: 14 in]
          }
          frame "---------- Lifeguard ----------" {
            n128 = Unbundle By Name(w371) -> ("Lifeguard"=w370:refnum<class "Lifeguard.lvclass">)
            n129 = Bundle By Name(cluster=w371, "Lifeguard"=w370) -> (w372:T5)
            n130 = call <vilib>:"Add State(s) to Queue__jki_lib_state_machine.vi"("State(s) in (\"\")"=w376) -> ("States Out"=w375:string)  [unwired: 14 in]
          }
          frame "Lifeguard: New Panels" {
            n131 = Unbundle By Name(w383) -> ("Lifeguard"=w381:refnum<class "Lifeguard.lvclass">, "Panels"=w382:T8)
            n132 = for {
              tunnel: w382 -> [w389] mode=indexing
              tunnel: [w388] -> w379 mode=indexing
              n133 = Unbundle By Name(w389) -> ("Control"=w388:refnum<vi>)
            }
            n134 = call "Lifeguard.NewPanels.vi"("error in (no error)"=w377, "New Panels"=w379, "Lifeguard"=w381) -> ("error out"=w378:errorcluster, "Lifeguard out"=w380:refnum<class "Lifeguard.lvclass">)  [unwired: 7 in]
            n135 = Bundle By Name(cluster=w383, "Lifeguard"=w380) -> (w384:T5)
            n136 = call <vilib>:"Add State(s) to Queue__jki_lib_state_machine.vi"("State(s) in (\"\")"=w387) -> ("States Out"=w386:string)  [unwired: 14 in]
          }
          frame "---------- Manager ----------" {
            n137 = Unbundle By Name(w391) -> ("Maui Manager"=w390:refnum<class "Maui Manager.lvclass">)
            n138 = Bundle By Name(cluster=w391, "Maui Manager"=w390) -> (w392:T5)
            n139 = call <vilib>:"Add State(s) to Queue__jki_lib_state_machine.vi"("State(s) in (\"\")"=w396) -> ("States Out"=w395:string)  [unwired: 14 in]
          }
          frame "Manager: Grey Rings" {
            n140 = Unbundle By Name(w401) -> ("Maui Manager"=w400:refnum<class "Maui Manager.lvclass">)
            n141 = call "GreyRings.vi"("error in (no error)"=w397, "Maui Manager in"=w400) -> ("error out"=w398:errorcluster, "Maui Manager out"=w399:refnum<class "Maui Manager.lvclass">)  [unwired: 8 in]
            n142 = Bundle By Name(cluster=w401, "Maui Manager"=w399) -> (w402:T5)
            n143 = call <vilib>:"Add State(s) to Queue__jki_lib_state_machine.vi"("State(s) in (\"\")"=w405) -> ("States Out"=w404:string)  [unwired: 14 in]
          }
          frame "Manager: Insert Subpanel" {
            n144 = Unbundle By Name(w412) -> ("Maui Manager"=w411:refnum<class "Maui Manager.lvclass">, "Panel"=w407:i32, "New Value"=w406:i32)
            n145 = call "InsertSubpanel.vi"("error in (no error)"=w408, "Subpanel"=w406, "Panel"=w407, "Maui Manager in"=w411) -> ("error out"=w409:errorcluster, "Maui Manager out"=w410:refnum<class "Maui Manager.lvclass">)  [unwired: 6 in]
            n146 = Bundle By Name(cluster=w412, "Maui Manager"=w410) -> (w413:T5)
            n147 = call <vilib>:"Add State(s) to Queue__jki_lib_state_machine.vi"("State(s) in (\"\")"=w416) -> ("States Out"=w415:string)  [unwired: 14 in]
          }
          frame "Manager: Initialize Panels" {
            n148 = Unbundle By Name(w421) -> ("Maui Manager"=w420:refnum<class "Maui Manager.lvclass">)
            n149 = call "InitializePanels.vi"("error in (no error)"=w417, "Maui Manager in"=w420) -> ("error out"=w418:errorcluster, "Maui Manager out"=w419:refnum<class "Maui Manager.lvclass">)  [unwired: 8 in]
            n150 = Bundle By Name(cluster=w421, "Maui Manager"=w419) -> (w422:T5)
            n151 = call <vilib>:"Add State(s) to Queue__jki_lib_state_machine.vi"("State(s) in (\"\")"=w425) -> ("States Out"=w424:string)  [unwired: 14 in]
          }
          frame "Manager: Set Subpanels" {
            n152 = Unbundle By Name(w433) -> ("Maui Manager"=w432:refnum<class "Maui Manager.lvclass">, "Subpanels"=w429:refnum<class "SMO.lvclass">[])
            n153 = call "Maui 2.0.GetProcesses.vi"("error in (no error)"=w426, "Subpanels"=w429) -> ("error out"=w427:errorcluster, "Processes"=w428:refnum<vi>[])  [unwired: 8 in]
            n154 = property class="Maui Manager.lvclass"(reference=w432, error in=w427, "Accessors:Processes"=w428) -> (reference out=w431:refnum<class "Maui Manager.lvclass">, error out=w430:errorcluster)
            n155 = Bundle By Name(cluster=w433, "Maui Manager"=w431) -> (w434:T5)
            n156 = call <vilib>:"Add State(s) to Queue__jki_lib_state_machine.vi"("State(s) in (\"\")"=w437) -> ("States Out"=w436:string)  [unwired: 14 in]
          }
          frame "Manager: Set Panels" {
            n157 = Unbundle By Name(w443) -> ("Maui Manager"=w442:refnum<class "Maui Manager.lvclass">, "Panels"=w440:T8)
            n158 = property class="Maui Manager.lvclass"(reference=w442, error in=w439, "Accessors:Panels"=w440) -> (reference out=w441:refnum<class "Maui Manager.lvclass">, error out=w438:errorcluster)
            n159 = Bundle By Name(cluster=w443, "Maui Manager"=w441) -> (w444:T5)
            n160 = call <vilib>:"Add State(s) to Queue__jki_lib_state_machine.vi"("State(s) in (\"\")"=w447) -> ("States Out"=w446:string)  [unwired: 14 in]
          }
        }
      }
    }
    frame Error {
    }
  }
  n161 = call-parent "Process.vi"("error in"=w8, "SMO"=w7) -> ("error out"=w5:errorcluster, "SMO out"=→"Maui 2.0 out":refnum<class "Maui 2.0.lvclass">)  [unwired: 8 in]
  n162 = Merge Errors(w5, w4) -> (→"error out":errorcluster)
